vi "Test RT Main API-RT.vi"() -> ()   [LabVIEW 2019]
doc: "RT Main API Tester for Real-Time."
uses:
  <vilib>/Utility/error.llb/DialogType.ctl
  RT Main.lvlib
panel:
  in  "Get Module Execution Status":bool
  in  "Exit":bool
  in  "Stop Module":bool
  in  "Run Module":bool
  out "error out":errorcluster
  out "last error":errorcluster
  out "Status":string
  out "Module Running?":bool
  # "This VI tests the API for the Module."
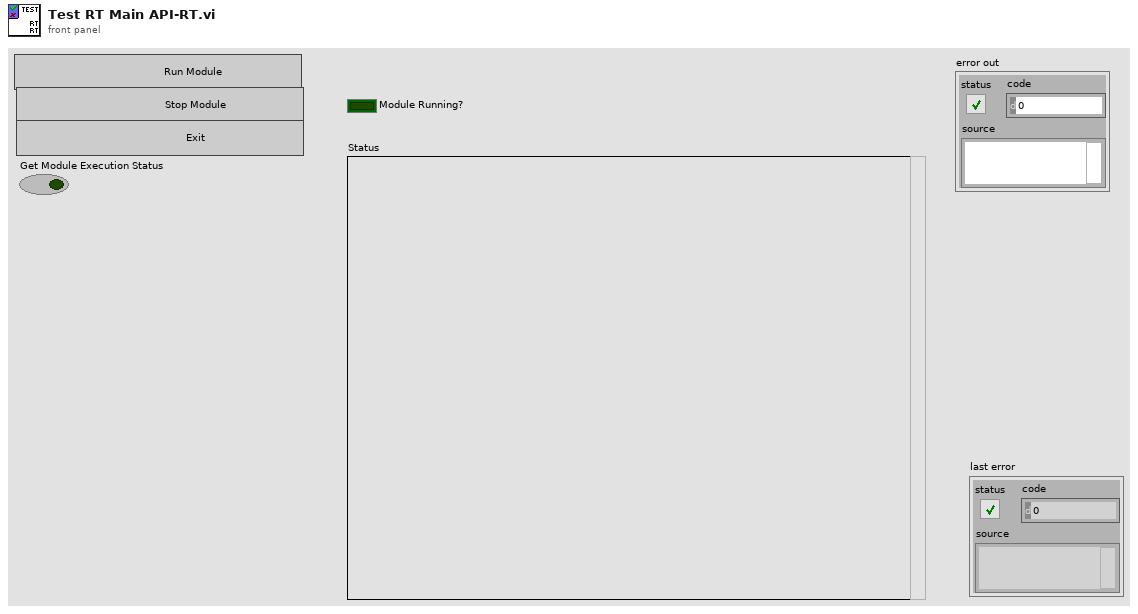
[diagram p1: front panel]
types:
  T1 = typedef "RT Main.lvlib/Broadcast Events--cluster.ctl" = cluster{"Module Did Init":refnum<user-event>, "Status Updated":refnum<user-event>, "Error Reported":refnum<user-event>, "Module Did Stop":refnum<user-event>, "Update Module Execution Status":refnum<user-event>}
  T2 = typedef "DialogType.ctl" = u16
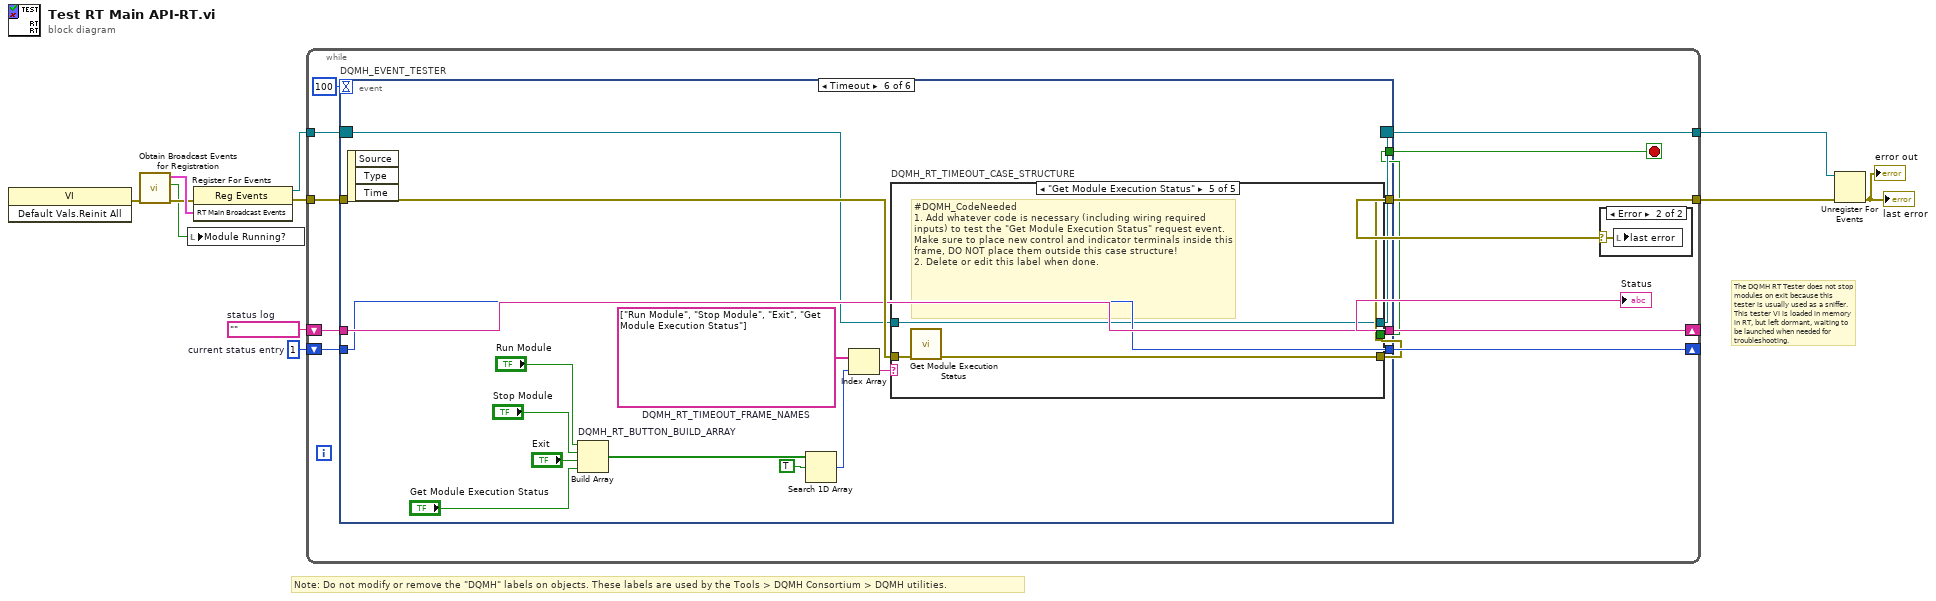
[diagram p0: block diagram]
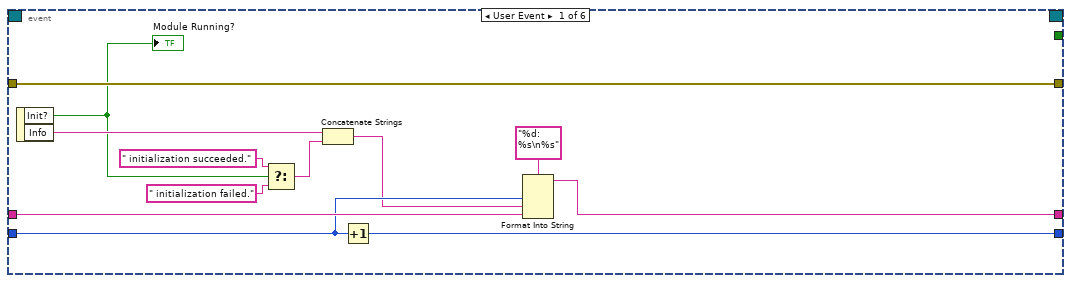
[diagram p3: hidden frame]
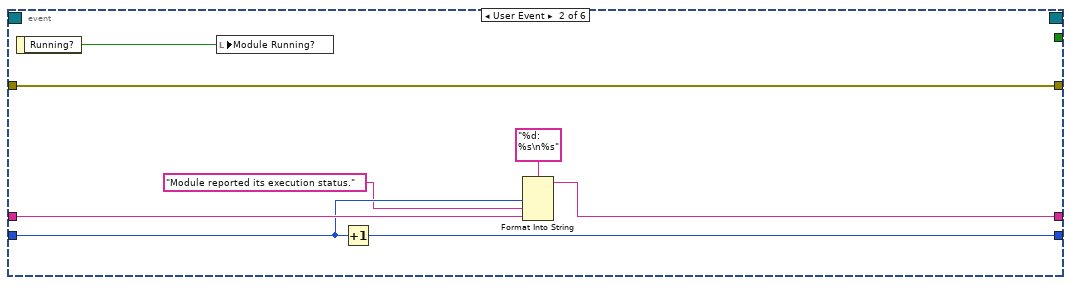
[diagram p4: hidden frame]
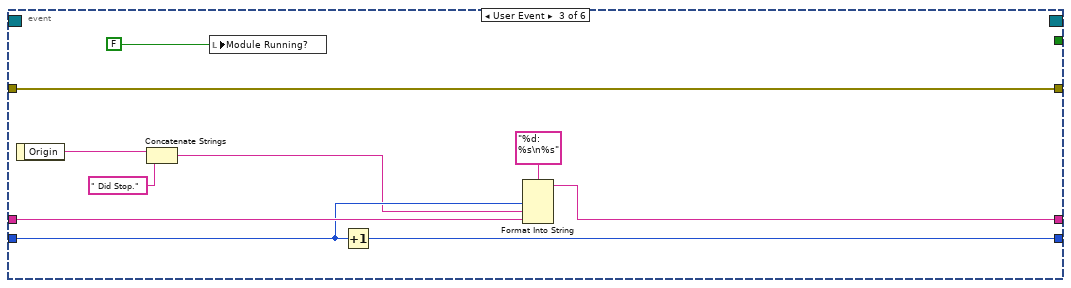
[diagram p5: hidden frame]
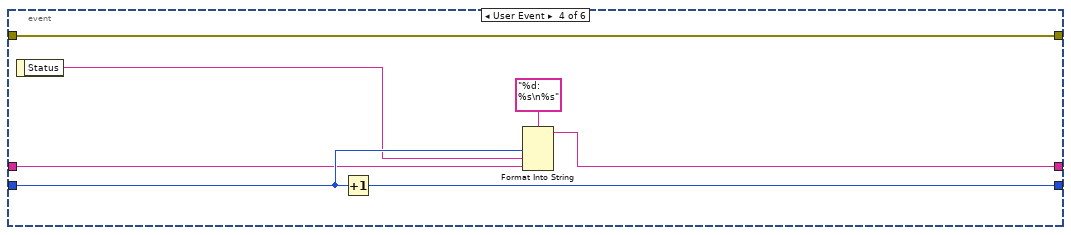
[diagram p6: hidden frame]
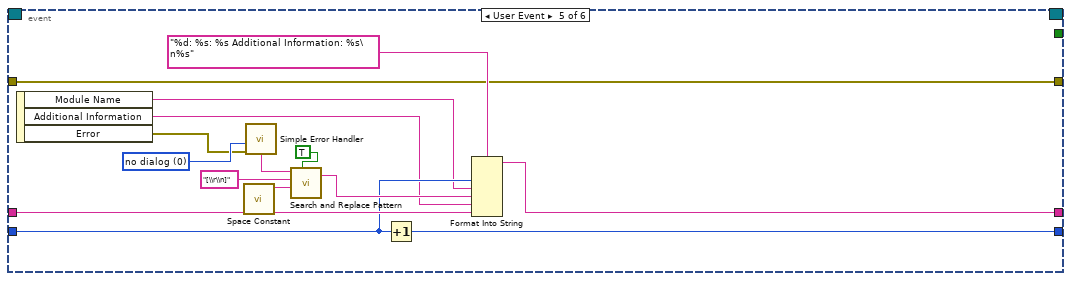
[diagram p7: hidden frame]
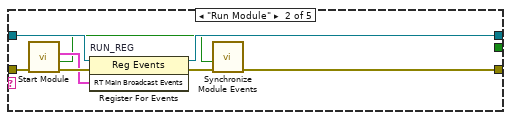
[diagram p9: hidden frame]
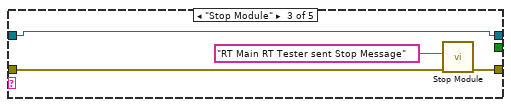
[diagram p10: hidden frame]
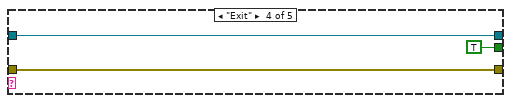
[diagram p11: hidden frame]
diagram:
  w10 = 1  # current status entry
  w11 = ""  # status log
  # "The DQMH RT Tester does not stop modules on exit because this tester is usually used as a sniffer. This tester VI is loaded in memory in RT, but left dormant, waiting to be launched when needed for troubleshooting."
  # "Note: Do not modify or remove the \"DQMH\" labels on objects. These labels are used by the Tools > DQMH Consortium > DQMH utilities."
  n1 = invoke class="VI" method="Default Vals.Reinit All"() -> (error out=w5:errorcluster)  [unwired: 3 in, 2 out]
  n2 = call "Obtain Broadcast Events for Registration.vi"("error in"=w5) -> ("error out"=w4:errorcluster, "Already running?"=w3:bool, "RT Main Broadcast Events"=w8:T1)  [unwired: 8 in]
  n3 = local write "Module Running?"(w3) -> ()
  n4 = register-events(error in=w4, w8) -> (reference out=w7:refnum<event-registration>, error out=w9:errorcluster)  [unwired: 1 in]
  n5 = while {
    tunnel: w7 -> [w21]
    tunnel: [w13] -> w2
    shift-right: [w17] -> _
    shift-left: w11 -> [w19]
    shift-right: [w18] -> _
    shift-left: w10 -> [w20]
    tunnel: w9 -> [w16]
    tunnel: [w15] -> w6
    stop <- w14 stop-if-true
    n6 = event "DQMH_EVENT_TESTER" shown="[5] Timeout" {
      selector: w21 -> [_ _ _ _ _ w86]
      dyn-events: [_ _ _ _ _ w85] -> w15
      timeout: 100 -> [_ _ _ _ _ _]
      tunnel: [_ _ _ _ _ w81] -> w14
      tunnel: [w34 w36 w43 w53 w63 w87] -> w13
      tunnel: w20 -> [w31 w40 w50 w56 w66 w88]
      tunnel: w19 -> [w32 w41 w51 w55 w67 w89]
      tunnel: [w29 w38 w48 w57 w65 w89] -> w17
      tunnel: [w30 w39 w49 w59 w64 w88] -> w18
      tunnel: w16 -> [w34 w36 w43 w53 w63 w90]
      event User Event {
        n7 = event-data() -> ("Init?"=w26:bool, "Info"=w28:string)  [unwired: 1 in]
        "Module Running?" <- w26
        n8 = Select(t=" initialization succeeded.", s=w26, f=" initialization failed.") -> (s? t:f=w23:string)
        n9 = Concatenate Strings(w28, w23) -> (w27:string)
        n10 = Increment(x=w31) -> (x+1=w30:i32)
        n11 = Format Into String(format string="%d: %s\n%s", w31, w27, w32) -> (resulting string=w29:string)  [unwired: 2 in, 1 out]
      }
      event User Event {
        n12 = event-data() -> ("Running?"=w35:bool)  [unwired: 1 in]
        n13 = local write "Module Running?"(w35) -> ()
        n14 = Increment(x=w40) -> (x+1=w39:i32)
        n15 = Format Into String(format string="%d: %s\n%s", w40, "Module reported its execution status.", w41) -> (resulting string=w38:string)  [unwired: 2 in, 1 out]
      }
      event User Event {
        n16 = event-data() -> ("Origin"=w47:string)  [unwired: 1 in]
        n17 = Concatenate Strings(w47, " Did Stop.") -> (w46:string)
        n18 = local write "Module Running?"(FALSE ("Module Did Init?")) -> ()
        n19 = Increment(x=w50) -> (x+1=w49:i32)
        n20 = Format Into String(format string="%d: %s\n%s", w50, w46, w51) -> (resulting string=w48:string)  [unwired: 2 in, 1 out]
      }
      event User Event {
        n21 = event-data() -> ("Status"=w54:string)  [unwired: 1 in]
        n22 = Increment(x=w56) -> (x+1=w59:i32)
        n23 = Format Into String(format string="%d: %s\n%s", w56, w54, w55) -> (resulting string=w57:string)  [unwired: 2 in, 1 out]
      }
      event User Event {
        w68 = T2 0 items=["no dialog", "OK message", "continue or stop message", "OK message + warnings", "continue/stop + warnings"] ("type of dialog (OK msg:1)")
        n24 = event-data() -> ("Module Name"=w62:string, "Additional Information"=w61:string, "Error"=w60:errorcluster)  [unwired: 1 in]
        n25 = call <vilib>:"Space Constant.vi"() -> ("String"=w72:string)
        n26 = call <vilib>:"Simple Error Handler.vi"("type of dialog (OK msg:1)"=w68, "error in (no error)"=w60) -> ("message"=w69:string)  [unwired: 3 in, 4 out]
        n27 = call <vilib>:"Search and Replace Pattern.vi"("string"=w69, "regular expression (\"\")"="[\\r\\n]" ("regular expression (\"\")"), "replace string (\"\")"=w72, "replace all? (F)"=TRUE ("replace all CR/LF with spaces")) -> ("result string"=w70:string)  [unwired: 1 in, 1 out]
        n28 = Increment(x=w66) -> (x+1=w64:i32)
        n29 = Format Into String(format string="%d: %s: %s Additional Information: %s\n%s", w66, w62, w70, w61, w67) -> (resulting string=w65:string)  [unwired: 2 in, 1 out]
      }
      event Timeout {
        w79 = string[] ["Run Module", "Stop Module", "Exit", "Get Module Execution Status"]  # DQMH_RT_TIMEOUT_FRAME_NAMES
        n30 = event-data() -> ()  [unwired: 1 in, 3 out]
        n31 = Build Array "DQMH_RT_BUTTON_BUILD_ARRAY"("Run Module", "Stop Module", "Exit", "Get Module Execution Status") -> (w76:bool[])
        n32 = Search 1D Array(1D array=w76, element=TRUE) -> (index of element=w78:i32)  [unwired: 1 in]
        n33 = Index Array(array=w79, index=w78) -> (element=w80:string)
        n34 = case "DQMH_RT_TIMEOUT_CASE_STRUCTURE" shown="\"Get Module Execution Status\"" w80 {
          tunnel: w90 -> [w92 w100 w103 w107 w110]
          tunnel: [w92 w94 w102 w107 w108] -> w87
          tunnel: w86 -> [w91 w98 w104 w106 w109]
          tunnel: [w91 w97 w104 w106 w109] -> w85
          tunnel: [_ _ _ TRUE _] -> w81
          frame "", Default {
          }
          frame "Run Module" {
            n35 = call "Start Module.vi"("error in"=w100) -> ("error out"=w96:errorcluster, "Wait for Event Sync?"=w93:bool, "RT Main Broadcast Events"=w95:T1)  [unwired: 6 in, 2 out]
            n36 = register-events "RUN_REG"(reference=w98, error in=w96, w95) -> (reference out=w97:refnum<event-registration>, error out=w99:errorcluster)
            n37 = call "Synchronize Module Events.vi"("error in"=w99, "Wait for Event Sync?"=w93) -> ("error out"=w94:errorcluster)  [unwired: 9 in]
          }
          frame "Stop Module" {
            n38 = call "Stop Module.vi"("error in"=w103, "Origin"="RT Main RT Tester sent Stop Message") -> ("error out"=w102:errorcluster)  [unwired: 9 in]
          }
          frame "Exit" {
          }
          frame "Get Module Execution Status" {
            # "#DQMH_CodeNeeded\n1. Add whatever code is necessary (including wiring required inputs) to test the \"Get Module Execution Status\" request event. Make sure to place new control and indicator terminals inside this frame, DO NOT place them outside this case structure!\n2. Delete or edit this label when done."
            n39 = call "Get Module Execution Status.vi"("error in"=w110) -> ("error out"=w108:errorcluster)  [unwired: 10 in]
          }
        }
      }
    }
    "Status" <- w17
    n40 = case shown="Error" w13 {
      selector: w13 -> [_ w22]
      frame No Error {
      }
      frame Error {
        n41 = local write "last error"(w22) -> ()
      }
    }
  }
  n42 = Unregister For Events(event registration refnum=w6, error in=w2) -> (error out=→"last error" →"error out":errorcluster)
